vi "FestoCPX.Valve(3out3in)_2.vi"(4 "Delay [ms] (0)":u32, 6 "Timeout [ms] (5000)":u32=5000, 8 "error in (no error)":errorcluster, 9 "Pos":i32, 10 "Valve outputs":T1[](array[typedef]), 11 "Inputs":T2[](array[typedef])) -> (0 "error out":errorcluster, 2 "Aborted?":bool, 3 "Timeout?":bool)   [LabVIEW 2016]
uses:
  FestoCPX.DI.Signal.ctl
  FestoCPX.DO.Signal.ctl
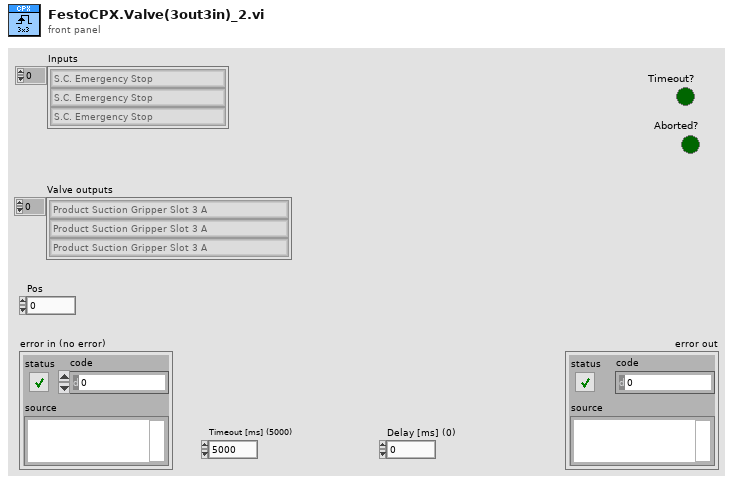
[diagram p1: front panel]
types:
  T1 = typedef "FestoCPX.DO.Signal.ctl" = enum16{"Safety Reset", "Air Main Valve", "Door Lock", "Button LED Start", "Button LED Stop", "Button LED Control", "Traffic LED Red", "Traffic LED Orange", "Traffic LED Green", "Horn", "Laser Interlock", "Laser Trigger", "Laser Fume Extractor", "Product Suction Gripper Slot 1 A", "Product Suction Gripper Slot 1 B", "Product Suction Gripper Slot 2 A", "Product Suction Gripper Slot 2 B", "Product Suction Gripper Slot 3 A", "Product Suction Gripper Slot 3 B", "Product Suction Gripper Slot 4 A", "Product Suction Gripper Slot 4 B", "Product Suction Gripper Final A", "Product Suction Gripper Final B", "Lamp", "Q1 Product Move Work", "Q1 Product Move Home", "Q2 Table Turn Work", "Q2 Table Turn Home", "Q3 Product Lift A", "Q3 Product Lift B", "Q4 Product Arm OK", "Q4 Product Arm NOK", "Q5 Product Arm Work", "Q6 Product BlowOut A", "Q6 Product BlowOut B"}
  T2 = typedef "FestoCPX.DI.Signal.ctl" = enum16{"S.C. Emergency Stop", "S.C. Side Door Close", "S.C. Front Door Close", "S.C. Front Door Secured", "Button Start", "Button Stop", "Button Control", "Product Move Home", "Product Move Work", "Table Position", "Table Lock", "Product Lift A Home", "Product Lift B Home", "Product Arm OK", "Product Arm NOK", "Product Arm Work", "Revolver ID 1", "Revolver ID 2", "Revolver ID 3", "Revolver ID 4", "Revolver ID 5", "Air Pressure Inside", "Air Pressure Inlet", "Product Slot 1 A Present", "Product Slot 1 B Present", "Product Slot 2 A Present", "Product Slot 2 B Present", "Product Slot 3 A Present", "Product Slot 3 B Present", "Product Slot 4 A Present", "Product Slot 4 B Present", "Product Final A Present", "Product Final B Present", "Product Output A Present", "Product Output B Present", "Product Container OK Present", "Product Container NOK Present", "Fork ID 1", "Fork ID 2"}
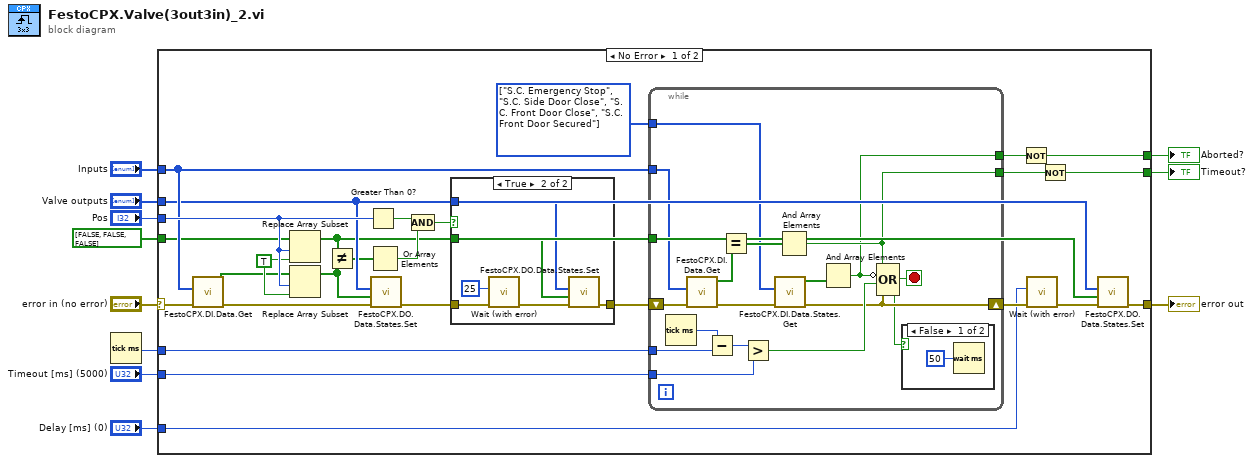
[diagram p0: block diagram]
diagram:
  n1 = Tick Count (ms)() -> (millisecond timer value=w7:u32)
  n2 = case shown="No Error" "error in (no error)" {
    selector: "error in (no error)" -> [w26 w63]
    tunnel: "Pos" -> [w27 _]
    tunnel: [w22 w63] -> w10
    tunnel: [w35 _] -> w9
    tunnel: w7 -> [w37 _]
    tunnel: "Timeout [ms] (5000)" -> [w36 _]
    tunnel: "Inputs" -> [w24 _]
    tunnel: "Valve outputs" -> [w21 _]
    tunnel: "Delay [ms] (0)" -> [w32 _]
    tunnel: [w28 _] -> w2
    tunnel: bool[] [FALSE, FALSE, FALSE] -> [w23 _]
    frame No Error {
      w18 = TRUE ("new element/subarray")
      w30 = T2[] [enum."S.C. Emergency Stop", enum."S.C. Side Door Close", enum."S.C. Front Door Close", enum."S.C. Front Door Secured"] items=["S.C. Emergency Stop", "S.C. Side Door Close", "S.C. Front Door Close", "S.C. Front Door Secured", "Button Start", "Button Stop", "Button Control", "Product Move Home", "Product Move Work", "Table Position", "Table Lock", "Product Lift A Home", "Product Lift B Home", "Product Arm OK", "Product Arm NOK", "Product Arm Work", "Revolver ID 1", "Revolver ID 2", "Revolver ID 3", "Revolver ID 4", "Revolver ID 5", "Air Pressure Inside", "Air Pressure Inlet", "Product Slot 1 A Present", "Product Slot 1 B Present", "Product Slot 2 A Present", "Product Slot 2 B Present", "Product Slot 3 A Present", "Product Slot 3 B Present", "Product Slot 4 A Present", "Product Slot 4 B Present", "Product Final A Present", "Product Final B Present", "Product Output A Present", "Product Output B Present", "Product Container OK Present", "Product Container NOK Present", "Fork ID 1", "Fork ID 2"] ("CPX.DI")
      n3 = call-poly "FestoCPX.DI.Data.Get.vi"("error in (no error)"=w26, "CPX.DI"=w24) -> ("error out"=w25:errorcluster, "State"=w12:bool[])  [unwired: 5 in, 3 out]
      n4 = Replace Array Subset(array=w23, new element=w18, index=w27) -> (w13:bool[])
      n5 = Replace Array Subset(array=w12, new element=w18, index=w27) -> (w19:bool[])
      n6 = Not Equal?(x=w13, y=w19) -> (x != y?=w17:bool[])
      n7 = Greater Than 0?(x=w27) -> (x > 0?=w14:bool)
      n8 = Or Array Elements(Boolean array=w17) -> (logical OR=w16:bool)
      n9 = call "FestoCPX.DO.Data.States.Set.vi"("error in (no error)"=w25, "State"=w19, "CPX.DO"=w21) -> ("error out"=w20:errorcluster)  [unwired: 8 in]
      n10 = Compound Arithmetic op=AND(w14, w16) -> (w15:bool)
      n11 = case shown="True" w15 {
        tunnel: [w38 w44] -> w31
        tunnel: w21 -> [_ w43]
        tunnel: w20 -> [w38 w42]
        tunnel: w13 -> [_ w39]
        frame False {
        }
        frame True {
          n12 = call "Wait (with error).vi"("error in (no error)"=w42, "milliseconds to wait"=u32 25) -> ("error out"=w41:errorcluster)  [unwired: 8 in, 1 out]
          n13 = call "FestoCPX.DO.Data.States.Set.vi"("error in (no error)"=w41, "State"=w39, "CPX.DO"=w43) -> ("error out"=w44:errorcluster)  [unwired: 8 in]
        }
      }
      n14 = while {
        shift-right: [w50] -> w33
        shift-left: w31 -> [w61]
        tunnel: w24 -> [w60]
        tunnel: [w53] -> w34
        tunnel: w37 -> [w58]
        tunnel: w36 -> [w56]
        tunnel: w13 -> [w55]
        tunnel: w30 -> [w49]
        tunnel: [w48] -> w29
        stop <- w47 stop-if-true
        n15 = Tick Count (ms)() -> (millisecond timer value=w59:u32)
        n16 = call-poly "FestoCPX.DI.Data.Get.vi"("error in (no error)"=w61, "CPX.DI"=w60) -> ("error out"=w51:errorcluster, "State"=w46:bool[])  [unwired: 5 in, 3 out]
        n17 = Subtract(x=w59, y=w58) -> (x-y=w57:u32)
        n18 = Equal?(x=w55, y=w46) -> (x = y?=w54:bool[])
        n19 = Greater?(x=w57, y=w56) -> (0:w52:bool)
        n20 = call "FestoCPX.DI.Data.States.Get.vi"("error in (no error)"=w51, "CPX.DI"=w49) -> ("error out"=w50:errorcluster, "State"=w45:bool[])  [unwired: 5 in, 3 out]
        n21 = And Array Elements(Boolean array=w54) -> (logical AND=w53:bool)
        n22 = And Array Elements(Boolean array=w45) -> (logical AND=w48:bool)
        n23 = Compound Arithmetic op=OR(w53, invert w48, w52, w50) -> (w47:bool)
        n24 = case shown="False" w47 {
          frame False {
            n25 = Wait (ms)(milliseconds to wait=u32 50) -> ()  [unwired: 1 out]
          }
          frame True {
          }
        }
      }
      n26 = Not(x=w29) -> (.not. x?=w28:bool)
      n27 = call "Wait (with error).vi"("error in (no error)"=w33, "milliseconds to wait"=w32) -> ("error out"=w22:errorcluster)  [unwired: 8 in, 1 out]
      n28 = Not(x=w34) -> (.not. x?=w35:bool)
      n29 = call "FestoCPX.DO.Data.States.Set.vi"("error in (no error)"=w22, "State"=w13, "CPX.DO"=w21) -> ()  [unwired: 8 in, 1 out]
    }
    frame Error {
    }
  }
  "error out" <- w10
  "Timeout?" <- w9
  "Aborted?" <- w2
